vi "Delete Step.vi"(8 "Error In":errorcluster, 10 "Index":i32, 11 "reference in":refnum<class "Recipe.lvclass">) -> (0 "Error Out":errorcluster, 3 "reference out":refnum<class "Recipe.lvclass">)   [LabVIEW 2021, in "Recipe.lvclass"]
uses:
  Recipe.lvclass
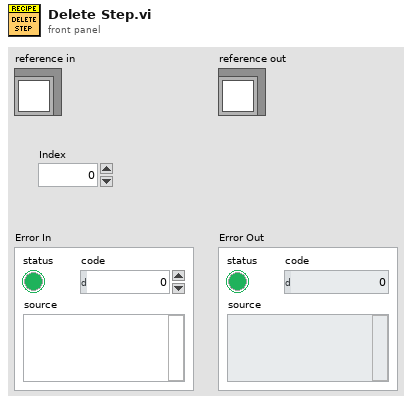
[diagram p1: front panel]
types:
  T1 = typedef "Recipe.lvclass/ObjectAttributes.ctl" = cluster{"Steps":refnum<class "Recipe Step.lvclass">[], "Current Info":cluster{"Current Index":u64}}
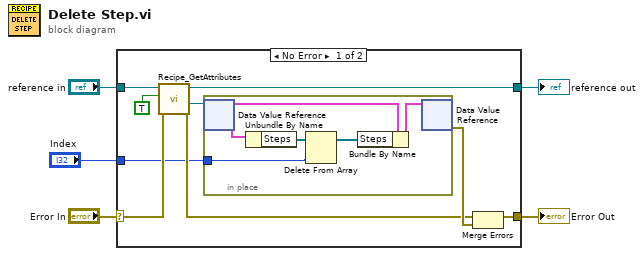
[diagram p0: block diagram]
diagram:
  n1 = case shown="No Error" "Error In" {
    selector: "Error In" -> [w13 w21]
    tunnel: [w10 w21] -> w4
    tunnel: [w11 w20] -> w2
    tunnel: "reference in" -> [w14 w20]
    tunnel: "Index" -> [w6 _]
    frame No Error {
      n2 = call "Recipe_GetAttributes.vi"("Error In"=w13, "OnlyGetDvrReference(False)"=TRUE, "reference in"=w14) -> ("Error Out"=w8:errorcluster, "DataRef"=w9:refnum<data-value>, "reference out"=w11:refnum<class "Recipe.lvclass">)  [unwired: 5 in, 1 out]
      n3 = in-place {
        in-place-border: w6 -> [w15]
        n4 = in-place-dvr #1(w9) -> (w18:T1)  [unwired: 1 out]
        n5 = Unbundle By Name(w18) -> ("Steps"=w17:refnum<class "Recipe Step.lvclass">[])
        n6 = Delete From Array(array=w17, index=w15) -> (array with subset deleted=w16:refnum<class "Recipe Step.lvclass">[])  [unwired: 1 in, 1 out]
        n7 = Bundle By Name(cluster=w18, "Steps"=w16) -> (w19:T1)
        n8 = in-place-dvr #1(w19) -> (w12:errorcluster)  [unwired: 1 out]
      }
      n9 = Merge Errors(w8, w12) -> (w10:errorcluster)
    }
    frame Error {
    }
  }
  "Error Out" <- w4
  "reference out" <- w2
